vi "StateDiagramPlugins_GetStates_txt.vi"(1 "Path":path=path "C:/Documents and Settings/Micke/Mina dokument/LabView/StateMachines/String1/StateString1.vi", 5 "error in (no error)":errorcluster) -> (15 "States":T1[](array[typedef]), 19 "error out":errorcluster)   [LabVIEW 2010]
uses:
  ReversedEngineering/ReversedEngineering StateMachineStateInfo.ctl
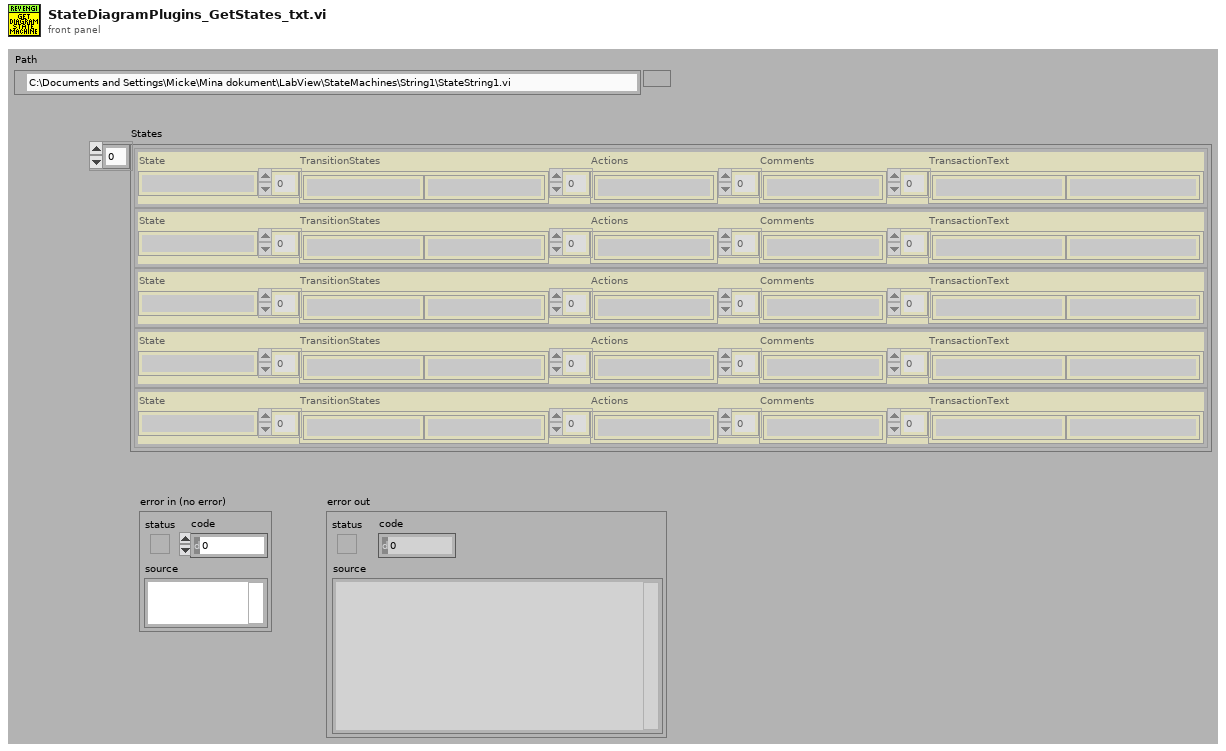
[diagram p1: front panel]
types:
  T1 = typedef "ReversedEngineering StateMachineStateInfo.ctl" = cluster{"State":string, "TransitionStates":string[], "Actions":string[], "Comments":string[], "TransactionText":string[]}
  T2 = cluster{"State":string, "TransitionStates":string[], "Actions":string[]}[]
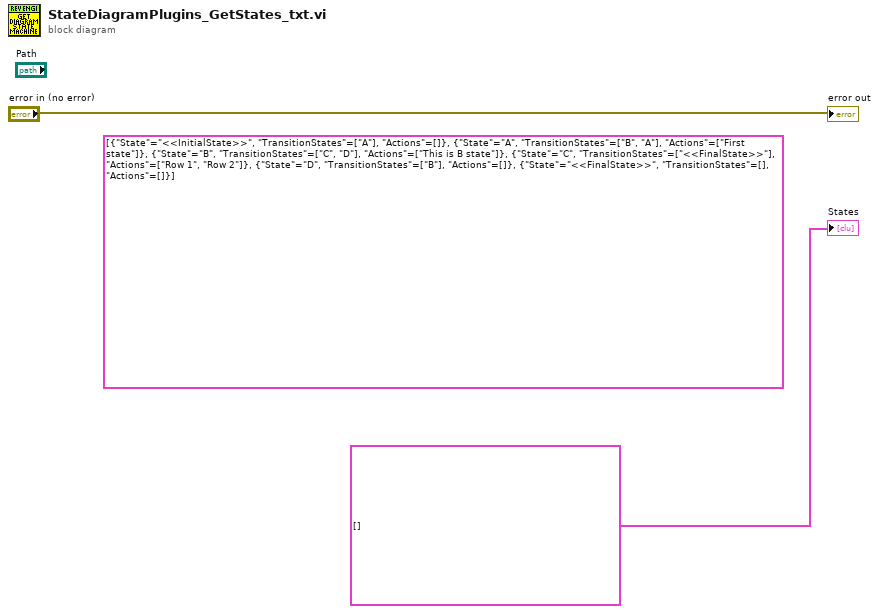
[diagram p0: block diagram]
diagram:
  (unwired) T2 [{"State"="<<InitialState>>", "TransitionStates"=["A"], "Actions"=[]}, {"State"="A", "TransitionStates"=["B", "A"], "Actions"=["First state"]}, {"State"="B", "TransitionStates"=["C", "D"], "Actions"=["This is B state"]}, {"State"="C", "TransitionStates"=["<<FinalState>>"], "Actions"=["Row 1", "Row 2"]}, {"State"="D", "TransitionStates"=["B"], "Actions"=[]}, {"State"="<<FinalState>>", "TransitionStates"=[], "Actions"=[]}] ("States")
  "error out" <- "error in (no error)"
  "States" <- T1[] [] ("States")
